vi "Write Camera ID.vi"(8 "error in (no error)":errorcluster, 10 "Camera ID":i32, 11 "Orca-Flash 4.0 V2 in":refnum<class "Orca-Flash 4.0 V2.lvclass">) -> (0 "error out":errorcluster, 3 "Orca-Flash 4.0 V2 out":refnum<class "Orca-Flash 4.0 V2.lvclass">)   [LabVIEW 2015]
uses:
  Orca-Flash 4.0 V2.lvclass
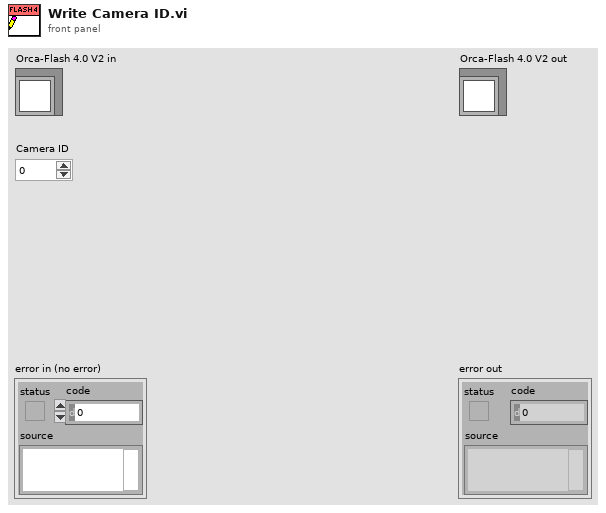
[diagram p1: front panel]
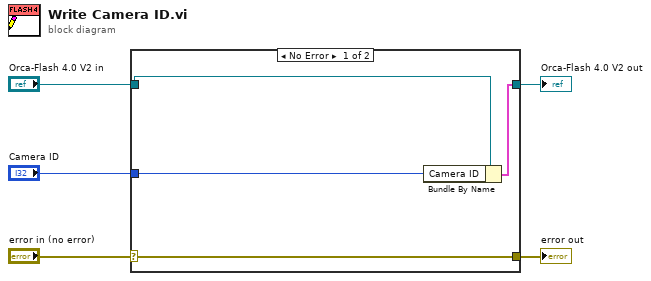
[diagram p0: block diagram]
diagram:
  n1 = case shown="No Error" "error in (no error)" {
    selector: "error in (no error)" -> [w9 w10]
    tunnel: [w9 w10] -> w4
    tunnel: [w7 w11] -> w2
    tunnel: "Orca-Flash 4.0 V2 in" -> [w8 w11]
    tunnel: "Camera ID" -> [w6 _]
    frame No Error {
      n2 = Bundle By Name(cluster=w8, "Camera ID"=w6) -> (w7:cluster{})
    }
    frame Error {
    }
  }
  "error out" <- w4
  "Orca-Flash 4.0 V2 out" <- w2
